vi "FPGA Independent SAR and DSA.vi"() -> ()   [LabVIEW 2025]
uses:
  <vilib>/Platform/TimedLoop/XDataNode/timing_clust.ctl
  <vilib>/Platform/TimedLoop/XDataNode/nitl_modes.ctl
  <vilib>/Platform/TimedLoop/XDataNode/wakeup.ctl
  <vilib>/LabVIEW Targets/FPGA/cRIO/shared/nicrio_ModuleControls/nicrio_cRIO-9234_DataRatesRing2.ctl
  <vilib>/rvi/Emulation/niFpgaGetClockAttributes.vi
  <vilib>/rvi/Emulation/niFpgaSctlEmulationGetInTimedLoop.vi
  <vilib>/rvi/Emulation/niFpgaEmulationReportErrorSimple.vi
  <vilib>/rvi/eio/common/nirviEmuTemplateMethod_errors.vi
  <vilib>/rvi/Emulation/niFpgaCriticalErrorInLSC.vi
  <vilib>/rvi/eio/common/nirviEmuTemplatePropertySet_noerrors.vi
  <vilib>/eio/EIONode/EIONode.xnode
  <vilib>/eio/EIOPropertyNode/EIOPropertyNode.xnode
  <vilib>/platform/TimedLoop/XDataNode/XDataNode.xnode
  <vilib>/rvi/eio/common/nirviEmuTemplatePropertyGet_errors.vi
  <vilib>/rvi/eio/common/nirviEmuTemplatePropertyGet_noerrors.vi
  <vilib>/rvi/eio/common/nirviEmuTemplatePropertySet_errors.vi
  <vilib>/Platform/TimedLoop/XDataNode/XDNodeRunTimeDep.lvlib
panel:
  out "Mod2/DIO3":bool
  out "Mod2/DIO2":bool
  out "Mod2/DIO1":bool
  out "Mod2/DIO0":bool
  in  "stop Fast Digital":bool
  in  "Mod1/DO3":bool
  in  "Mod1/DO2":bool
  in  "Mod1/DO1":bool
  in  "Mod1/DO0":bool
  in  "stop Slow Digital":bool
  out "DSA Data":fxp<+/-,24,4>[](array[numeric])
  in  "stop DSA":bool
  out "SAR Data":fxp<+/-,26,5>[](array[numeric])
  in  "stop SAR":bool
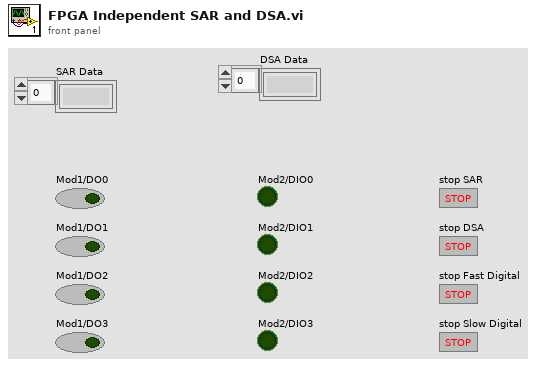
[diagram p1: front panel]
types:
  T1 = typedef "nicrio_cRIO-9234_DataRatesRing2.ctl" = u8
  T2 = typedef "XDNodeRunTimeDep.lvlib/timing_clust.ctl" = cluster{"Expected End [f-1]":u64, "Actual End [f-1]":u64, "Finished Late? [f-1]":bool, "Expected End [i-1]":u64, "Actual End [i-1]":u64, "Finished Late? [i-1]":bool, "Expected Start [i]":u64, "Actual Start [i]":u64, "Expected Start [f]":u64, "Actual Start [f]":u64, "Source Name":string, "Structure Name":string, "Period":i64, "Deadline":i64, "Offset":i64, "Start":i64, "Priority":i32, "Timeout":i32, "Mode":T3, "Wakeup Reason":T4, "Error":errorcluster, "Source Type":string, "Secondary Source Type":string, "Global End Time":u64, "Global Start Time":u64, "Frame Duration":u64, "Iteration Duration":u64, "Assigned CPU":i32, "I/O Scan Engine Mode":u32}
  T3 = typedef "XDNodeRunTimeDep.lvlib/nitl_modes.ctl" = enum32{"No Change", "Process missed periods, maintain original phase", "Discard missed periods, maintain original phase", "Process missed periods, ignore original phase", "Discard missed periods, ignore original phase"}
  T4 = typedef "XDNodeRunTimeDep.lvlib/wakeup.ctl" = enum32{"Normal", "Aborted", "Asynchronous wakeup", "Timing source error", "Timed loop error", "Timeout"}
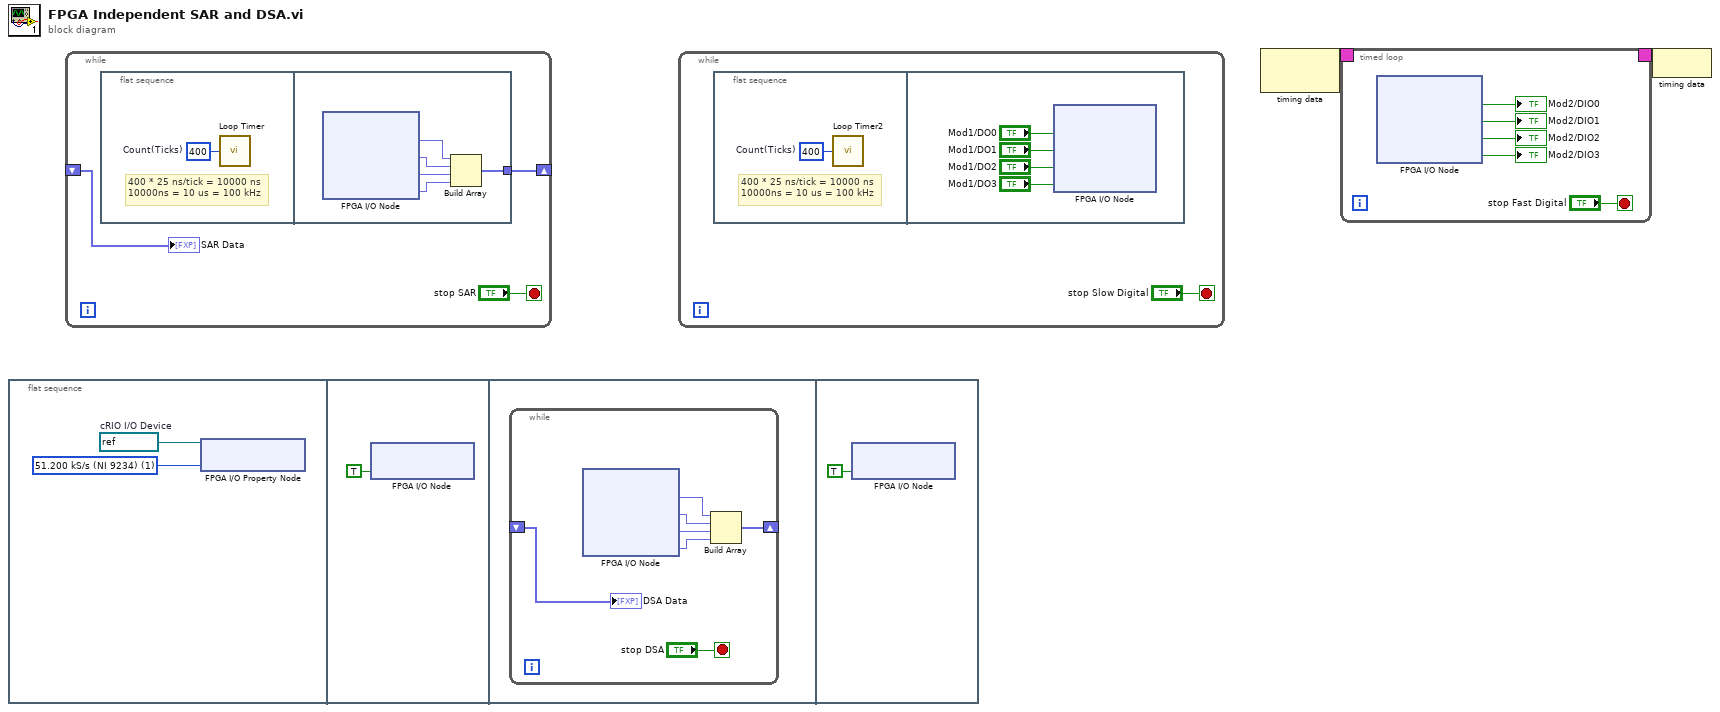
[diagram p0: block diagram]
diagram:
  n1 = flat-sequence {
    frame #0 {
      w3 = T1 1 items=["51.200 kS/s (NI 9234)"=1, "25.600 kS/s (NI 9234)"=2, "17.067 kS/s (NI 9234)"=3, "12.800 kS/s (NI 9234)"=4, "10.240 kS/s (NI 9234)"=5, "8.533 kS/s (NI 9234)"=6, "7.314 kS/s (NI 9234)"=7, "6.400 kS/s (NI 9234)"=8, "5.689 kS/s (NI 9234)"=9, "5.120 kS/s (NI 9234)"=10, "4.654 kS/s (NI 9234)"=11, "4.267 kS/s (NI 9234)"=12, "3.938 kS/s (NI 9234)"=13, "3.657 kS/s (NI 9234)"=14, "3.413 kS/s (NI 9234)"=15, "3.200 kS/s (NI 9234)"=16, "3.012 kS/s (NI 9234)"=17, "2.845 kS/s (NI 9234)"=18, "2.695 kS/s (NI 9234)"=19, "2.560 kS/s (NI 9234)"=20, "2.438 kS/s (NI 9234)"=21, "2.328 kS/s (NI 9234)"=22, "2.226 kS/s (NI 9234)"=23, "2.133 kS/s (NI 9234)"=24, "2.048 kS/s (NI 9234)"=25, "1.969 kS/s (NI 9234)"=26, "1.896 kS/s (NI 9234)"=27, "1.829 kS/s (NI 9234)"=28, "1.765 kS/s (NI 9234)"=29, "1.707 kS/s (NI 9234)"=30, "1.652 kS/s (NI 9234)"=31] ("Data Rate")
      w4 = refnum<k21> "Mod7"  # cRIO I/O Device
      n2 = xnode "FPGA I/O Property Node"("FPGA I/O In"=w4, "Data Rate"=w3) -> ()  [unwired: 1 out]
    }
    frame #1 {
      n3 = xnode "FPGA I/O Node"("Mod7/Start"=TRUE) -> ()  [unwired: 1 in, 1 out]
    }
    frame #2 {
      n4 = while {
        shift-right: [w11] -> _
        shift-left: _ -> [w10]
        stop <- "stop DSA" stop-if-true
        n5 = xnode "FPGA I/O Node"() -> ("Mod7/AI0"=w9:fxp<+/-,24,4>, "Mod7/AI1"=w8:fxp<+/-,24,4>, "Mod7/AI2"=w7:fxp<+/-,24,4>, "Mod7/AI3"=w6:fxp<+/-,24,4>)  [unwired: 4 in, 4 out]
        n6 = Build Array(w9, w8, w7, w6) -> (w11:fxp<+/-,24,4>[])
        "DSA Data" <- w10
      }
    }
    frame #3 {
      n7 = xnode "FPGA I/O Node"("Mod7/Stop"=TRUE ("Mod7/Start")) -> ()  [unwired: 1 in, 1 out]
    }
  }
  n8 = while {
    shift-right: [w15] -> _
    shift-left: _ -> [w14]
    stop <- "stop SAR" stop-if-true
    n9 = flat-sequence {
      tunnel: [w18] -> w15
      frame #0 {
        w17 = u32 400  # Count(Ticks)
        # "400 * 25 ns/tick = 10000 ns\n10000ns = 10 us = 100 kHz"
        n10 = call "Loop Timer"("Count(Ticks)"=w17) -> ()  [unwired: 1 out]
      }
      frame #1 {
        n11 = xnode "FPGA I/O Node"() -> ("Mod4/AI0"=w22:fxp<+/-,26,5>, "Mod4/AI1"=w21:fxp<+/-,26,5>, "Mod4/AI2"=w20:fxp<+/-,26,5>, "Mod4/AI3"=w19:fxp<+/-,26,5>)  [unwired: 4 in, 4 out]
        n12 = Build Array(w22, w21, w20, w19) -> (w18:fxp<+/-,26,5>[])
      }
    }
    "SAR Data" <- w14
  }
  n13 = while {
    stop <- "stop Slow Digital" stop-if-true
    n14 = flat-sequence {
      frame #0 {
        w24 = u32 400  # Count(Ticks)
        # "400 * 25 ns/tick = 10000 ns\n10000ns = 10 us = 100 kHz"
        n15 = call "Loop Timer2"("Count(Ticks)"=w24) -> ()  [unwired: 1 out]
      }
      frame #1 {
        n16 = xnode "FPGA I/O Node"("Mod1/DO0"="Mod1/DO0", "Mod1/DO1"="Mod1/DO1", "Mod1/DO2"="Mod1/DO2", "Mod1/DO3"="Mod1/DO3") -> ()  [unwired: 4 in, 4 out]
      }
    }
  }
  n17 = node-c288() -> (w2:T2)  [unwired: 1 in]
  n18 = timed-loop {
    timing: w2 -> [_]
    timing-out: [_] -> w1
    stop <- "stop Fast Digital" stop-if-true
    n19 = xnode "FPGA I/O Node"() -> ("Mod2/DIO0"=→"Mod2/DIO0":bool, "Mod2/DIO1"=→"Mod2/DIO1":bool, "Mod2/DIO2"=→"Mod2/DIO2":bool, "Mod2/DIO3"=→"Mod2/DIO3":bool)  [unwired: 4 in, 4 out]
  }
  n20 = node-c288(w1) -> ()
